vi "clearWFMQueue.vi"(8 "error in (no error)":errorcluster, 11 "DAQmx in":refnum<class "DAQmx.lvclass">) -> (0 "error out":errorcluster, 3 "DAQmx out":refnum<class "DAQmx.lvclass">)   [LabVIEW 2019, in "DAQmx.lvclass"]
uses:
  DAQmx.lvclass
  DAQmx.lvclass/DAQmx.ctl
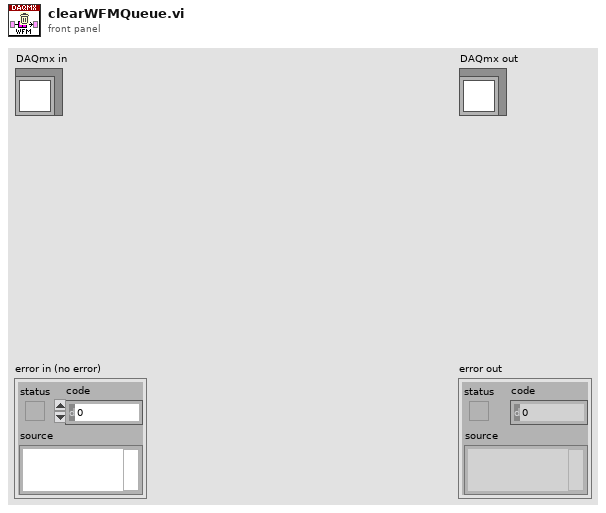
[diagram p1: front panel]
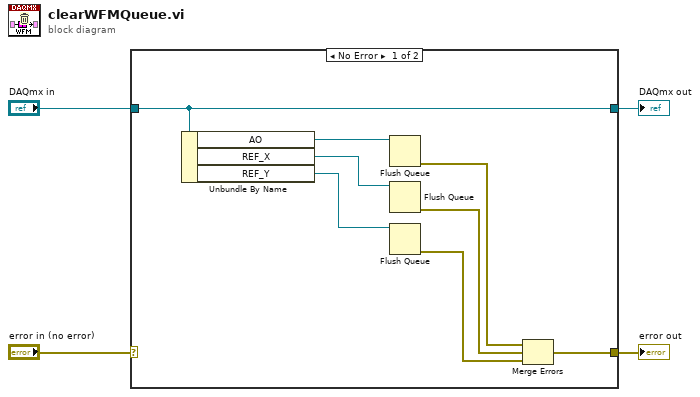
[diagram p0: block diagram]
diagram:
  n1 = case shown="No Error" "error in (no error)" {
    selector: "error in (no error)" -> [_ w14]
    tunnel: [w8 w14] -> w3
    tunnel: [w12 w13] -> w1
    tunnel: "DAQmx in" -> [w12 w13]
    frame No Error {
      n2 = Unbundle By Name(w12) -> ("AO"=w11:refnum<queue>, "REF_X"=w10:refnum<queue>, "REF_Y"=w9:refnum<queue>)
      n3 = Flush Queue(queue=w11) -> (error out=w5:errorcluster)  [unwired: 1 in, 2 out]
      n4 = Flush Queue(queue=w10) -> (error out=w6:errorcluster)  [unwired: 1 in, 2 out]
      n5 = Flush Queue(queue=w9) -> (error out=w7:errorcluster)  [unwired: 1 in, 2 out]
      n6 = Merge Errors(w5, w6, w7) -> (w8:errorcluster)
    }
    frame Error {
    }
  }
  "error out" <- w3
  "DAQmx out" <- w1
